vi "GetAvailRessGen.vi"(8 "ErrorIn(No Error)":errorcluster caption="entrée d'erreur (pas d'erreur)", 11 "VI reference":refnum<vi> caption="référence au VI") -> (0 "sortie d'erreur":errorcluster, 3 "ResArray":string[][](array[string]))   [LabVIEW 2019]
uses:
  <vilib>/Instr/_visa.llb/VISA Find Search Mode.ctl
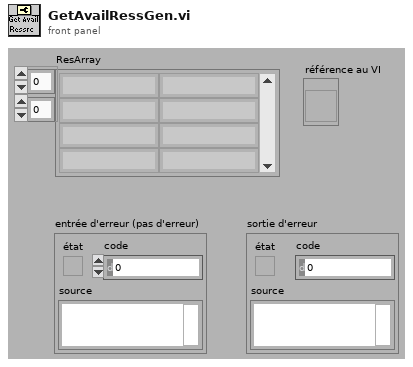
[diagram p1: front panel]
types:
  T1 = enum32{"Invalid", "Standard", "Closed", "Hidden", "Minimized", "Maximized"}[]
  T2 = typedef "VISA Find Search Mode.ctl" = u32
  T3 = enum32{"Invalid", "Standard", "Closed", "Hidden", "Minimized", "Maximized"}
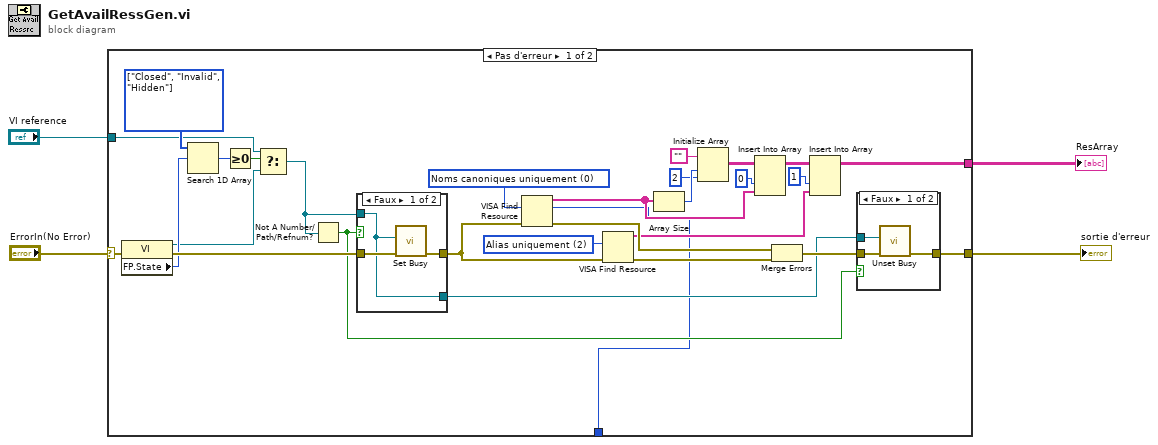
[diagram p0: block diagram]
diagram:
  n1 = case shown="Pas d'erreur" "ErrorIn(No Error)" {
    selector: "ErrorIn(No Error)" -> [w15 w42]
    tunnel: [w18 w42] -> w3
    tunnel: [w20 _] -> w2
    tunnel: "VI reference" -> [w8 _]
    tunnel: [w5 _] -> _
    frame No Error {
      w11 = T1 [enum."Closed", enum."Invalid", enum."Hidden"] items=["Invalid", "Standard", "Closed", "Hidden", "Minimized", "Maximized"]
      w30 = T2 2 items=["Noms canoniques uniquement"=0, "Alias uniquement"=2, "Inclure les alias correspondants"=3, "Inclure tous les alias"=4] ("Search Mode")
      w31 = T2 0 items=["Noms canoniques uniquement"=0, "Alias uniquement"=2, "Inclure les alias correspondants"=3, "Inclure tous les alias"=4] ("Search Mode")
      n2 = property class="VI"(error in=w15) -> (reference out=w7:refnum<vi>, error out=w14:errorcluster, "FP.State"=w12:T3)  [unwired: 1 in]
      n3 = Search 1D Array(1D array=w11, element=w12) -> (index of element=w10:i32)  [unwired: 1 in]
      n4 = Greater Or Equal To 0?(x=w10) -> (x >= 0?=w9:bool)
      n5 = Select(t=w8, s=w9, f=w7) -> (s? t:f=w6:refnum<vi>)
      n6 = Not A Number/Path/Refnum?(number/path/refnum=w6) -> (NaN/Path/Refnum?=w13:bool)
      n7 = case shown="Faux" w13 {
        tunnel: [w40 w41] -> w19
        tunnel: [w38 _] -> w16
        tunnel: w14 -> [w39 w41]
        tunnel: w6 -> [w38 _]
        frame False {
          n8 = call <vilib>:"Set Busy.vi"("error in (no error)"=w39, "VI reference (current VI)"=w38) -> ("error out"=w40:errorcluster)  [unwired: 8 in, 1 out]
        }
        frame True {
        }
      }
      n9 = VISA Find Resource(8:w19, 10:w31) -> (0:w32:errorcluster, 2:w5:u32, 3:w21:string[])  [unwired: 1 in]
      n10 = VISA Find Resource(8:w19, 10:w30) -> (0:w33:errorcluster, 3:w24:string[])  [unwired: 1 in, 1 out]
      n11 = Array Size(array=w21) -> (size(s)=w23:i32)
      n12 = Initialize Array("", w23, 2 ("taille de la dimension")) -> (w28:string[][])
      n13 = Insert Into Array(array=w28, index (col)=0 ("indice"), new element=w21) -> (w26:string[][])  [unwired: 1 in]
      n14 = Merge Errors(w32, w33) -> (w17:errorcluster)
      n15 = Insert Into Array(array=w26, index (col)=1 ("indice"), new element=w24) -> (w20:string[][])  [unwired: 1 in]
      n16 = case shown="Faux" w13 {
        tunnel: [w36 w37] -> w18
        tunnel: w17 -> [w35 w37]
        tunnel: w16 -> [w34 _]
        frame False {
          n17 = call <vilib>:"Unset Busy.vi"("error in (no error)"=w35, "VI reference (current VI)"=w34) -> ("error out"=w36:errorcluster)  [unwired: 9 in]
        }
        frame True {
        }
      }
    }
    frame Error {
    }
  }
  "sortie d'erreur" <- w3
  "ResArray" <- w2
